vi "Cypher XY LVDT Parameters_Asylum.vi"() -> ()   [LabVIEW 2016]
panel:
  in  "Cypher YLVDT Offset":dbl=-1.24
  in  "Cypher XLVDT Offset":dbl=0.9
  in  "Cypher YLVDT Sens":dbl=4.80459e-06
  in  "Cypher XLVDT Sens":dbl=4.99773e-06
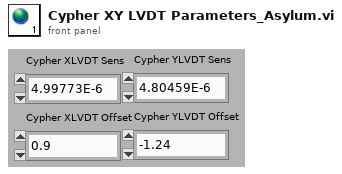
[diagram p1: front panel]
diagram:
